vi "Auton1.vi"(10 "Shoot distance (ft)":dbl, 11 "Distance from tape (ft)":dbl) -> ()   [LabVIEW 2013]
uses:
  <vilib>/Rock Robotics/WPI/Solenoid/WPI_SolenoidValue.ctl
  Device Refrences.vi
  <vilib>/Rock Robotics/WPI/Solenoid/WPI_SolenoidSetEnum.vi
  Robot Global Data.vi
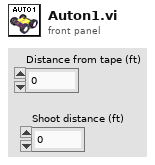
[diagram p1: front panel]
types:
  T1 = typedef "WPI_SolenoidValue.ctl" = enum16{"Off", "On", "Forward", "Reverse"}
  T2 = cluster{"proportional gain (Kc)":dbl, "integral time (Ti, min)":dbl, "derivative time (Td, min)":dbl}
  T3 = typedef "WPI_EncoderDevRef.ctl" = cluster{"DevStatus":errorcluster, "EncoderIndex":T4, "CounterIndex":T5, "DistancePerCount":dbl, "Decoding Type":T6}
  T4 = typedef "FPGA_EncoderIdx.ctl" = enum8{"Enc 0", "Enc 1", "Enc 2", "Enc 3", "Invalid"}
  T5 = typedef "FPGA_CounterCtrSystemIndex.ctl" = enum8{"Ctr 0", "Ctr 1", "Ctr 2", "Ctr 3", "Ctr 4", "Ctr 5", "Ctr 6", "Ctr 7", "Invalid"}
  T6 = typedef "WPI_EncoderType.ctl" = enum16{"1x", "2x", "4x"}
  T7 = cluster{"Compressor running":bool, "Compressor enabled":bool, "Right Encoder":dbl, "Left Encoder":dbl, "Ultrasonic Sensor":dbl, "Light Sensor":dbl}
  T8 = typedef "WPI_RobotDriveDevRef.ctl" = cluster{"DevStatus":errorcluster, "Motors[]":T9[], "Square Inputs":bool, "Max Output":dbl, "Isochronous":bool}
  T9 = typedef "WPI_MotorControlDeviceRef.ctl" = cluster{"DeviceStatus":errorcluster, "Type":enum16{"PWM", "CAN"}, "PWM":cluster{"Digital Module":T10, "PWM Channel":T11, "DeadBand":T12}, "CAN":cluster{"Device Number":u8, "Control Mode":T13, "Semaphore":T14, "Max Vout":dbl}, "Invert":bool, "TransformRef":T15, "InvTransformRef":T15}
  T10 = typedef "FPGA_TypedefDigitalModule.ctl" = enum16{"Digital Module 1", "Digital Module 2"}
  T11 = typedef "FPGA_DIOPWMChannel.ctl" = enum8{"PWM 1", "PWM 2", "PWM 3", "PWM 4", "PWM 5", "PWM 6", "PWM 7", "PWM 8", "PWM 9", "PWM 10", "Invalid"}
  T12 = typedef "WPI_PWMDeadband.ctl" = cluster{"Name":string, "maxPositivePwm":i32, "minPositivePwm":i32, "centerPwm":i32, "maxNegativePwm":i32, "minNegativePwm":i32, "angularRange":u16}
  T13 = typedef "WPI_CANJaguar_ControlMode.ctl" = enum8{"Percent VBus", "Current", "Speed", "Position", "Voltage"}
  T14 = typedef "Semaphore RefNum" = refnum<k1>
  T15 = typedef "WPI_PWMTransform_ConPane.ctl" = refnum<vi>
  T16 = cluster{"Drive Output Values":dbl[], "Shooter Solenoid":T1, "Pickup Solenoid":T1, "Pickup Motor":dbl}
  T17 = typedef "WPI_SolenoidDevRef.ctl" = cluster{"DevStatus":errorcluster, "Solenoid Module":T18, "Forward Solenoid Channel":T19, "Reverse Solenoid Channel":T19}
  T18 = typedef "FPGA_TypedefSolenoidModule.ctl" = enum16{"Solenoid Module 1", "Solenoid Module 2"}
  T19 = typedef "WPI_SolenoidChannel.ctl" = enum8{"Solenoid 1", "Solenoid 2", "Solenoid 3", "Solenoid 4", "Solenoid 5", "Solenoid 6", "Solenoid 7", "Solenoid 8", "Invalid"}
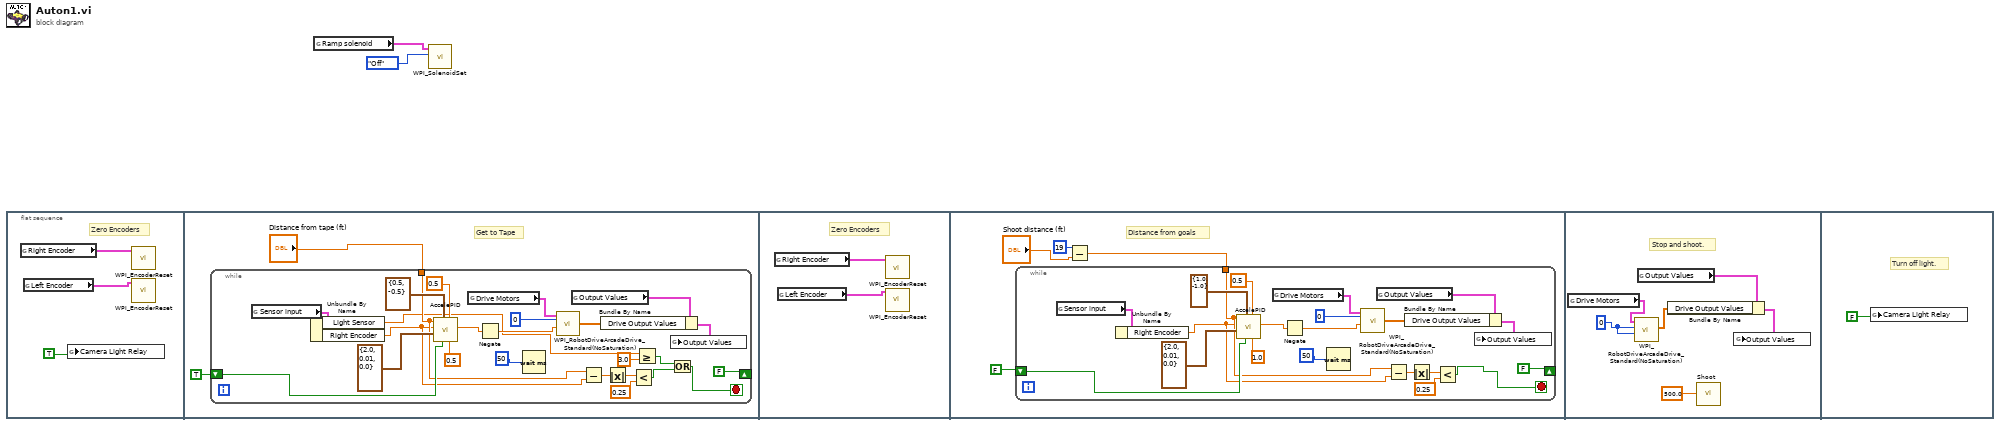
[diagram p0: block diagram]
diagram:
  n1 = flat-sequence {
    frame #0 {
      # "Zero Encoders"
      n2 = global read "Device Refrences.vi" "Right Encoder"() -> (w4:T3)
      n3 = global read "Device Refrences.vi" "Left Encoder"() -> (w5:T3)
      n4 = global write "Robot Global Data.vi" "Camera Light Relay"(TRUE) -> ()
      n5 = call <vilib>:"WPI_EncoderReset.vi"("EncoderDevRef"=w4) -> ()  [unwired: 9 in, 2 out]
      n6 = call <vilib>:"WPI_EncoderReset.vi"("EncoderDevRef"=w5) -> ()  [unwired: 9 in, 2 out]
    }
    frame #1 {
      # "Get to Tape"
      n7 = while {
        tunnel: "Distance from tape (ft)" -> [w19]
        shift-right: [FALSE] -> _
        shift-left: TRUE -> [w27]
        stop <- w11 stop-if-true
        n8 = global read "Robot Global Data.vi" "Sensor input"() -> (w29:T7)
        n9 = Unbundle By Name(w29) -> ("Light Sensor"=w10:dbl, "Right Encoder"=w18:dbl)
        n10 = call "AccelePID.vi"("Top Speed"=0.5 ("Acceleration Rate"), "Acceleration Rate"=0.5, "reinitialize? (F)"=w27, "output range"=cluster{"output high":dbl, "output low":dbl} {"output high"=0.5, "output low"=-0.5}, "PID gains"=T2 {"proportional gain (Kc)"=2.0, "integral time (Ti, min)"=0.01, "derivative time (Td, min)"=0.0}, "process variable"=w18, "setpoint"=w19) -> ("output"=w14:dbl)  [unwired: 3 in, 1 out]
        n11 = global read "Device Refrences.vi" "Drive Motors"() -> (w25:T8)
        n12 = Negate(x=w14) -> (-x=w13:dbl)
        n13 = Wait (ms)(milliseconds to wait=50) -> ()  [unwired: 1 out]
        n14 = call <vilib>:"WPI_RobotDriveArcadeDrive_Standard(NoSaturation).vi"("Y axis value"=w13, "X axis value"=0, "RobotDriveDevRef"=w25) -> ("Motor Values"=w22:dbl[])  [unwired: 1 in, 7 out]
        n15 = global read "Robot Global Data.vi" "Output Values"() -> (w23:T16)
        n16 = Subtract(x=w19, y=w18) -> (x-y=w17:dbl)
        n17 = Bundle By Name(cluster=w23, "Drive Output Values"=w22) -> (w21:T16)
        n18 = Absolute Value(x=w17) -> (abs(x)=w16:dbl)
        n19 = Less?(x=w16, y=0.25) -> (x < y?=w12:bool)
        n20 = Greater Or Equal?(x=w10, y=3.0) -> (x >= y?=w8:bool)
        n21 = global write "Robot Global Data.vi" "Output Values"(w21) -> ()
        n22 = Or(x=w8, y=w12) -> (x .or. y?=w11:bool)
      }
    }
    frame #2 {
      # "Zero Encoders"
      n23 = global read "Device Refrences.vi" "Right Encoder"() -> (w34:T3)
      n24 = global read "Device Refrences.vi" "Left Encoder"() -> (w33:T3)
      n25 = call <vilib>:"WPI_EncoderReset.vi"("EncoderDevRef"=w34) -> ()  [unwired: 9 in, 2 out]
      n26 = call <vilib>:"WPI_EncoderReset.vi"("EncoderDevRef"=w33) -> ()  [unwired: 9 in, 2 out]
    }
    frame #3 {
      # "Distance from goals"
      n27 = Subtract(x=19, y="Shoot distance (ft)") -> (x-y=w35:dbl)
      n28 = while {
        tunnel: w35 -> [w46]
        shift-right: [FALSE] -> _
        shift-left: FALSE -> [w54]
        stop <- w39 stop-if-true
        n29 = global read "Robot Global Data.vi" "Sensor input"() -> (w56:T7)
        n30 = Unbundle By Name(w56) -> ("Right Encoder"=w45:dbl)
        n31 = call "AccelePID.vi"("Top Speed"=1.0 ("Acceleration Rate"), "Acceleration Rate"=0.5, "reinitialize? (F)"=w54, "output range"=cluster{"output high":dbl, "output low":dbl} {"output high"=1.0, "output low"=-1.0}, "PID gains"=T2 {"proportional gain (Kc)"=2.0, "integral time (Ti, min)"=0.01, "derivative time (Td, min)"=0.0}, "process variable"=w45, "setpoint"=w46) -> ("output"=w41:dbl)  [unwired: 3 in, 1 out]
        n32 = global read "Device Refrences.vi" "Drive Motors"() -> (w52:T8)
        n33 = Negate(x=w41) -> (-x=w40:dbl)
        n34 = Wait (ms)(milliseconds to wait=50) -> ()  [unwired: 1 out]
        n35 = call <vilib>:"WPI_RobotDriveArcadeDrive_Standard(NoSaturation).vi"("Y axis value"=w40, "X axis value"=0, "RobotDriveDevRef"=w52) -> ("Motor Values"=w49:dbl[])  [unwired: 1 in, 7 out]
        n36 = global read "Robot Global Data.vi" "Output Values"() -> (w50:T16)
        n37 = Subtract(x=w46, y=w45) -> (x-y=w44:dbl)
        n38 = Bundle By Name(cluster=w50, "Drive Output Values"=w49) -> (w48:T16)
        n39 = Absolute Value(x=w44) -> (abs(x)=w43:dbl)
        n40 = Less?(x=w43, y=0.25) -> (x < y?=w39:bool)
        n41 = global write "Robot Global Data.vi" "Output Values"(w48) -> ()
      }
    }
    frame #4 {
      w61 = 0
      # "Stop and shoot."
      n42 = global read "Device Refrences.vi" "Drive Motors"() -> (w62:T8)
      n43 = call <vilib>:"WPI_RobotDriveArcadeDrive_Standard(NoSaturation).vi"("Y axis value"=w61, "X axis value"=w61, "RobotDriveDevRef"=w62) -> ("Motor Values"=w63:dbl[])  [unwired: 1 in, 7 out]
      n44 = global read "Robot Global Data.vi" "Output Values"() -> (w65:T16)
      n45 = Bundle By Name(cluster=w65, "Drive Output Values"=w63) -> (w64:T16)
      n46 = call "Shoot.vi"("Duration"=500.0) -> ()  [unwired: 11 in]
      n47 = global write "Robot Global Data.vi" "Output Values"(w64) -> ()
    }
    frame #5 {
      # "Turn off light."
      n48 = global write "Robot Global Data.vi" "Camera Light Relay"(FALSE) -> ()
    }
  }
  n49 = global read "Device Refrences.vi" "Ramp solenoid"() -> (w2:T17)
  n50 = call-poly <vilib>:"WPI_SolenoidSet.vi"("Value"=WPI_SolenoidValue."Off", "SolenoidDevRef"=w2) -> ()  [unwired: 8 in, 2 out]
